vi "Read constructors.vi"(9 "PythonConverter_GUI in":refnum<class "PythonConverter_GUI.lvclass">) -> (3 "PythonConverter_GUI out":refnum<class "PythonConverter_GUI.lvclass">, 4 "constructors":variant)   [LabVIEW 2014, in "Raspberry Pi Compatible Compiler for LabVIEW.lvlib" / "PythonConverter_GUI.lvclass"]
uses:
  PythonConverter_GUI.lvclass
  PythonConverter_GUI.lvclass/PythonConverter_GUI.ctl
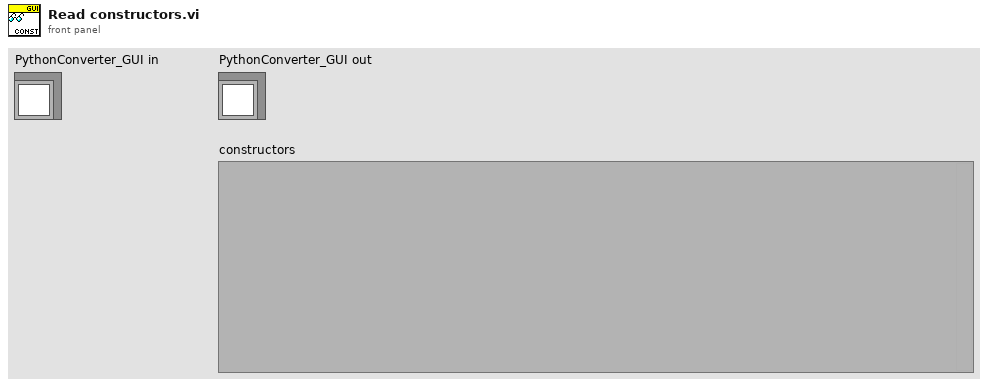
[diagram p1: front panel]
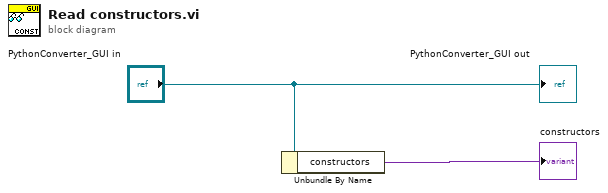
[diagram p0: block diagram]
diagram:
  n1 = Unbundle By Name("PythonConverter_GUI in") -> ("constructors"=→"constructors":variant)
  "PythonConverter_GUI out" <- "PythonConverter_GUI in"
